vi "test_vlp_udp-comm.vi"() -> ()   [LabVIEW 2019]
panel:
  in  "OnboardPC IP":string="223.171.56.43"
  out "LiDAR Image Gray":T1(plugin-control)
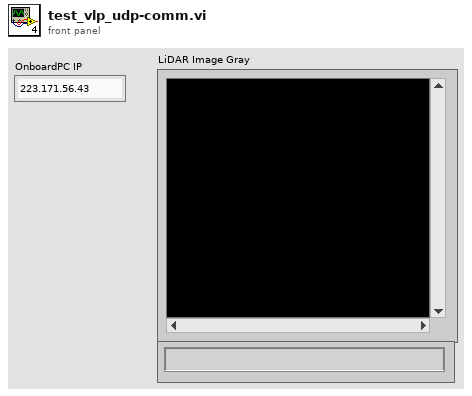
[diagram p1: front panel]
types:
  T1 = typedef "IMAQ Image.ctl" = refnum<image>
  T2 = typedef "Image Type" = u32
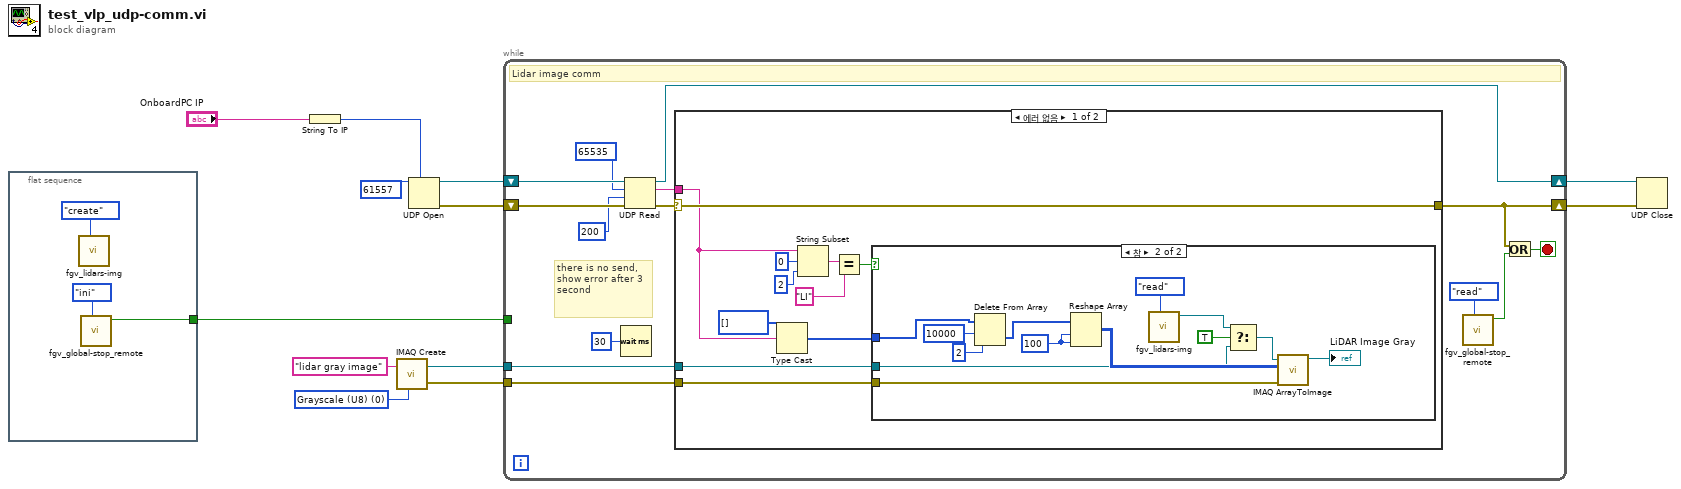
[diagram p0: block diagram]
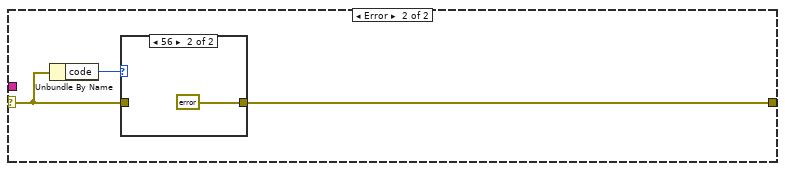
[diagram p3: hidden frame]
diagram:
  w6 = T2 0 items=["Grayscale (U8)", "Grayscale (I16)", "Grayscale (SGL)", "Complex (CSG)", "RGB (U32)", "HSL (U32)", "RGB (U64)", "Grayscale (U16)"] ("Image Type")
  n1 = flat-sequence {
    tunnel: [w14] -> w1
    frame #0 {
      n2 = call "fgv_lidars-img.vi"("cmd"=enum16{"create", "read", "close"}."create") -> ()  [unwired: 10 in, 1 out]
      n3 = call "fgv_global-stop_remote.vi"("cmd"=enum16{"ini", "read", "stop"}."ini") -> ("stop status"=w14:bool)  [unwired: 10 in]
    }
  }
  n4 = String To IP(1:"OnboardPC IP") -> (0:w2:u32)
  n5 = call "IMAQ Create"("Image Name"="lidar gray image", "Image Type"=w6) -> ("New Image"=w4:T1, "error out"=w5:errorcluster)  [unwired: 3 in]
  n6 = UDP Open(7:w2, 11:u16 61557 ("port")) -> (port=w12:refnum<k16>, 0:w11:errorcluster)  [unwired: 3 in, 1 out]
  n7 = while {
    shift-right: [w22] -> w10
    shift-left: w12 -> [w29]
    shift-right: [w21] -> w9
    shift-left: w11 -> [w28]
    tunnel: w4 -> [w20]
    tunnel: w5 -> [w19]
    tunnel: w1 -> [_]
    stop <- w25 stop-if-true
    # "there is no send, show error after 3 second"
    # "Lidar image comm"
    n8 = Wait (ms)(milliseconds to wait=u32 30) -> ()  [unwired: 1 out]
    n9 = UDP Read(connection ID=w29, max size (548)=65535, timeout ms (25000)=200, 8:w28) -> (data out=w27:string, error out=w23:errorcluster, 3:w22:refnum<k16>)  [unwired: 2 out]
    n10 = case shown="에러 없음" w23 {
      selector: w23 -> [w39 w56]
      tunnel: w27 -> [w32 _]
      tunnel: [w39 w54] -> w21
      tunnel: w20 -> [w38 _]
      tunnel: w19 -> [w37 _]
      frame No Error {
        n11 = Type Cast(type=u8[] [], x=w32) -> (*(type *) &x=w30:u8[])
        n12 = String Subset(string=w32, offset (0)=0, length (rest)=2 ("length (rest)")) -> (substring=w34:string)
        n13 = Equal?(x=w34, y="LI") -> (x = y?=w31:bool)
        n14 = case shown="참" w31 {
          tunnel: w30 -> [_ w53]
          tunnel: w38 -> [_ w44]
          tunnel: w37 -> [_ w49]
          frame False {
          }
          frame True {
            w51 = 100 ("dimension size")
            n15 = Delete From Array(array=w53, length=10000, index=2) -> (deleted portion=w46:u8[])  [unwired: 1 out]
            n16 = Reshape Array(w46, w51, w51) -> (w50:u8[][])
            n17 = call "fgv_lidars-img.vi"("cmd"=enum16{"create", "read", "close"}."read") -> ("New Image"=w42:T1)  [unwired: 10 in]
            n18 = Select(t=w42, s=TRUE, f=w44) -> (s? t:f=w43:T1)
            n19 = call "IMAQ ArrayToImage"("error in (no error)"=w49, "Image Pixels (U8)"=w50, "Image"=w43) -> ("Image Out"=→"LiDAR Image Gray":T1)  [unwired: 7 in, 1 out]
          }
        }
      }
      frame Error {
        n20 = Unbundle By Name(w56) -> ("code"=w55:i32)
        n21 = case shown="56" w55 {
          tunnel: w56 -> [w57 _]
          tunnel: [w57 errorcluster {"status"=FALSE, "code"=0, "source"=""} ("error IO")] -> w54
          frame 0, Default {
          }
          frame 56 {
          }
        }
      }
    }
    n22 = call "fgv_global-stop_remote.vi"("cmd"=enum16{"ini", "read", "stop"}."read") -> ("stop status"=w16:bool)  [unwired: 10 in]
    n23 = Or(x=w21, y=w16) -> (x .or. y?=w25:bool)
  }
  n24 = UDP Close(connection ID=w10, 8:w9) -> ()  [unwired: 2 out]
